vi "ReadCalibrationFromFile (SubVI).vi"(2 "Calibration file path":path, 7 "error in (no error)":errorcluster) -> (12 "Orientation":string, 13 "error out":errorcluster, 14 "Stave ID":string, 15 "User notes":string, 16 "CameraWD":dbl format="%#_13g", 17 "um/Pixel":dbl format="%#_13g", 18 "Angle":dbl format="%#_13g", 19 "Stave Origin":dbl[](array[numeric]))   [LabVIEW 2016]
uses:
  <vilib>/Utility/config.llb/Read Key (String).vi
  <vilib>/Utility/config.llb/Read Key (Double).vi
  <vilib>/Utility/config.llb/NI_LVConfig.lvlib
panel:
  # "General"
  # "Camera Calibration"
  # "Stave basis calibration"
  # "(Date and time recorded)"
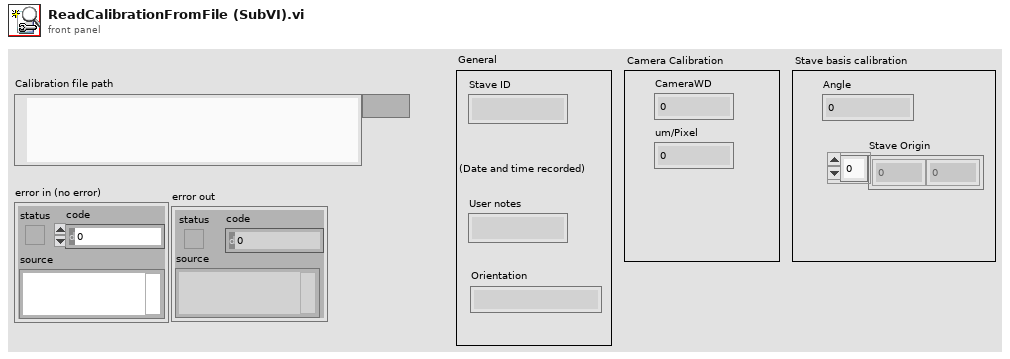
[diagram p1: front panel]
types:
  T1 = typedef "NI_LVConfig.lvlib/Config Data RefNum.ctl" = refnum<k1>
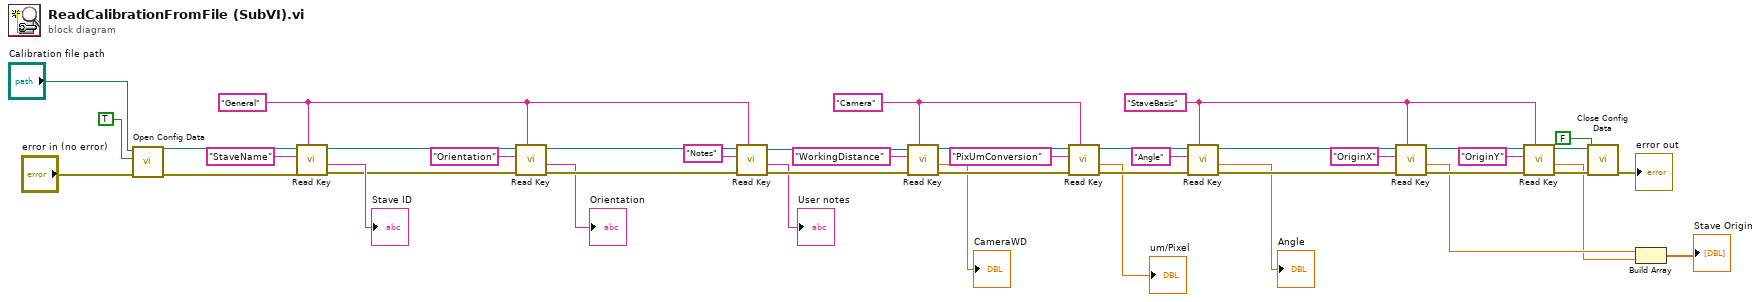
[diagram p0: block diagram]
diagram:
  w18 = "StaveBasis" ("section")
  w27 = "Camera" ("section")
  w5 = "General" ("section")
  n1 = call <vilib>:"Open Config Data.vi"("error in (no error)"="error in (no error)", "create file if necessary (T)"=TRUE, "configuration file path"="Calibration file path") -> ("error out"=w38:errorcluster, "refnum"=w40:T1)  [unwired: 6 in, 1 out]
  n2 = call-poly <vilib>:"Read Key.vi"("section"=w5, "error in (no error)"=w38, "key"="StaveName", "refnum"=w40) -> ("error out"=w3:errorcluster, "value"=→"Stave ID":string, "refnum out"=w7:T1)  [unwired: 4 in, 1 out]
  n3 = call-poly <vilib>:"Read Key.vi"("section"=w5, "error in (no error)"=w3, "key"="Orientation", "refnum"=w7) -> ("error out"=w2:errorcluster, "value"=→"Orientation":string, "refnum out"=w6:T1)  [unwired: 4 in, 1 out]
  n4 = call-poly <vilib>:"Read Key.vi"("section"=w5, "error in (no error)"=w2, "key"="Notes", "refnum"=w6) -> ("error out"=w29:errorcluster, "value"=→"User notes":string, "refnum out"=w28:T1)  [unwired: 4 in, 1 out]
  n5 = call-poly <vilib>:"Read Key.vi"("section"=w27, "error in (no error)"=w29, "key"="WorkingDistance", "refnum"=w28) -> ("error out"=w36:errorcluster, "value"=→"CameraWD":dbl, "refnum out"=w31:T1)  [unwired: 4 in, 1 out]
  n6 = call-poly <vilib>:"Read Key.vi"("section"=w27, "error in (no error)"=w36, "key"="PixUmConversion", "refnum"=w31) -> ("error out"=w35:errorcluster, "value"=→"um/Pixel":dbl, "refnum out"=w34:T1)  [unwired: 4 in, 1 out]
  n7 = call-poly <vilib>:"Read Key.vi"("section"=w18, "error in (no error)"=w35, "key"="Angle", "refnum"=w34) -> ("error out"=w24:errorcluster, "value"=→"Angle":dbl, "refnum out"=w21:T1)  [unwired: 4 in, 1 out]
  n8 = call-poly <vilib>:"Read Key.vi"("section"=w18, "error in (no error)"=w24, "key"="OriginX", "refnum"=w21) -> ("error out"=w23:errorcluster, "value"=w14:dbl, "refnum out"=w22:T1)  [unwired: 4 in, 1 out]
  n9 = call-poly <vilib>:"Read Key.vi"("section"=w18, "error in (no error)"=w23, "key"="OriginY", "refnum"=w22) -> ("error out"=w19:errorcluster, "value"=w13:dbl, "refnum out"=w20:T1)  [unwired: 4 in, 1 out]
  n10 = call <vilib>:"Close Config Data.vi"("error in (no error)"=w19, "write file if changed (T)"=FALSE, "refnum"=w20) -> ("error out"=→"error out":errorcluster)  [unwired: 7 in, 1 out]
  n11 = Build Array(w14, w13) -> (→"Stave Origin":dbl[])
